vi "SiRealCenterFinder2Circles.vi"() -> ()   [LabVIEW 2019]
uses:
  <vilib>/userDefined/High Color/IMAQdx.ctl
  Other Models/2010/Motion/AbortSingle.vi
  <vilib>/vision/NI_Vision_Development_Module.lvlib
panel:
  in  "AutoFocus":bool
  in  "InitialStepSize":dbl=0.1 format="%#_13g"
  in  "AbortAutoFocus":bool
  in  "VisibilityInCamera":enum16{"JoyStick", "ClickToMove", "AllVisible"}(ring)
  out "UsedCoordinates":string
  in  "AdjustCamera":T1={"+Y"=FALSE, "-Z"=FALSE, "Done"=FALSE, "+Z"=FALSE, "-Y"=FALSE, "-X"=FALSE, "+X"=FALSE, "MoveXYBy(mm)"=0.25, "MoveZBy(mm)"=0.1} {"MoveZBy(mm)" format="%#_13g"}
  in  "StopJoyStick":bool
  out "CameraGcode":string
  in  "SiOnBPFiducials":path=path "C:/Users/TTUHEP/Documents/LabVIEW/GantryPrograms/Configs/SiOnBPFiducialsA1.txt"
  out "Dev":dbl
  out "ImageCurrent":T2(plugin-control)
  out "Image2":T2(plugin-control)
  out "Image1":T2(plugin-control)
  out "Output XYZU":string
  in  "HexaboardEdges":path=path "C:/Users/TTUHEP/Documents/LabVIEW/GantryPrograms/Configs/PCB1_4Points.txt"
  in  "SiFiducials":path=path "C:/Users/TTUHEP/Documents/LabVIEW/GantryPrograms/Utilities/WorkInProgress/SensorFids4At30deg.txt"
  in  "Component":enum16{"Baseplate", "Si", "SiOnBP", "PCB"}(ring)=enum."Si"
  in  "BasePlateEdges":path=path "C:/Users/TTUHEP/Documents/LabVIEW/GantryPrograms/Configs/Baseplate1CuPoints.txt"
  # "Use \"Si\" or \"SiOnBP\".\nNot supported: \"Baseplate\", \"PCB\""
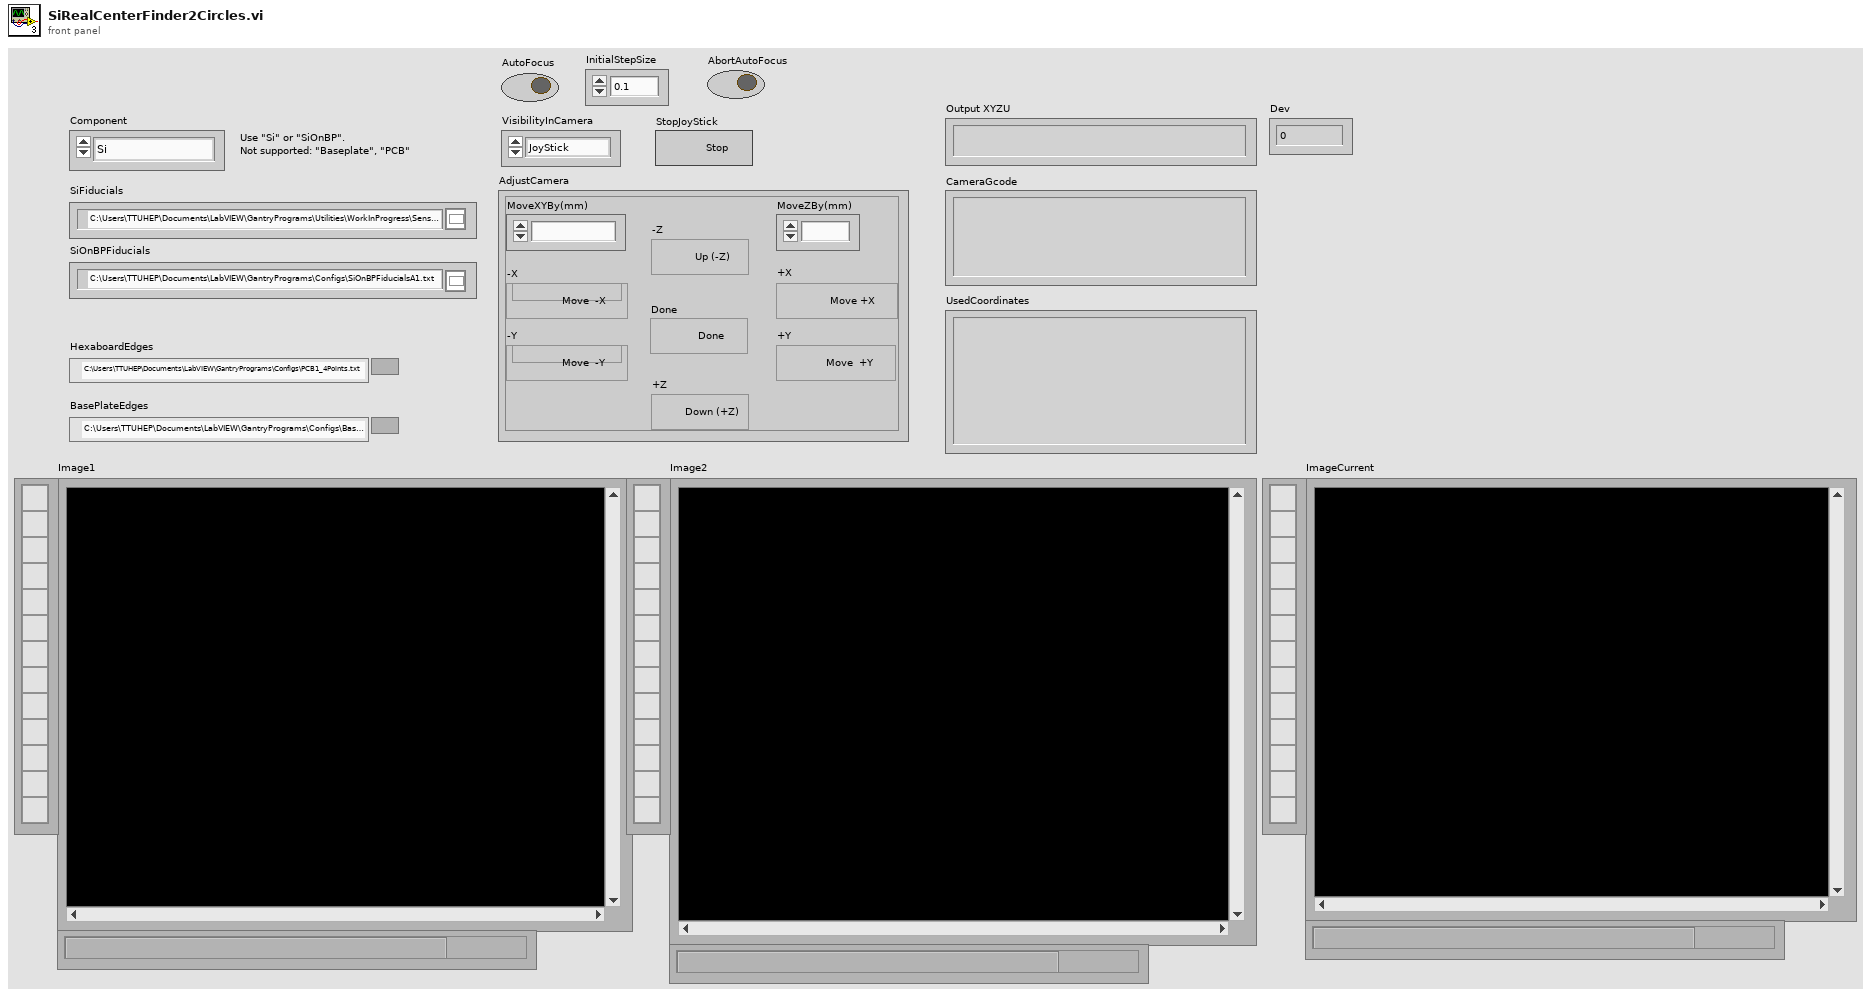
[diagram p1: front panel]
types:
  T1 = cluster{"+Y":bool, "-Z":bool, "Done":bool, "+Z":bool, "-Y":bool, "-X":bool, "+X":bool, "MoveXYBy(mm)":dbl, "MoveZBy(mm)":dbl}
  T2 = typedef "IMAQ Image.ctl" = refnum<image>
  T3 = typedef "IMAQdx.ctl" = refnum<k21>
  T4 = enum16{"Convolution", "Differentiation", "Gradient", "Prewitt", "Roberts", "Sigma", "Sobel"}
  T5 = typedef "Image Type" = u32
  T6 = cluster{"Position":cluster{"X":sgl, "Y":sgl}, "Radius":dbl, "Score":dbl}
  T7 = enum16{"Left Button", "Center Button", "Right Button", "Window Close"}
  T8 = enum16{"open", "replace", "create", "open or create", "replace or create", "replace or create with confirmation"}
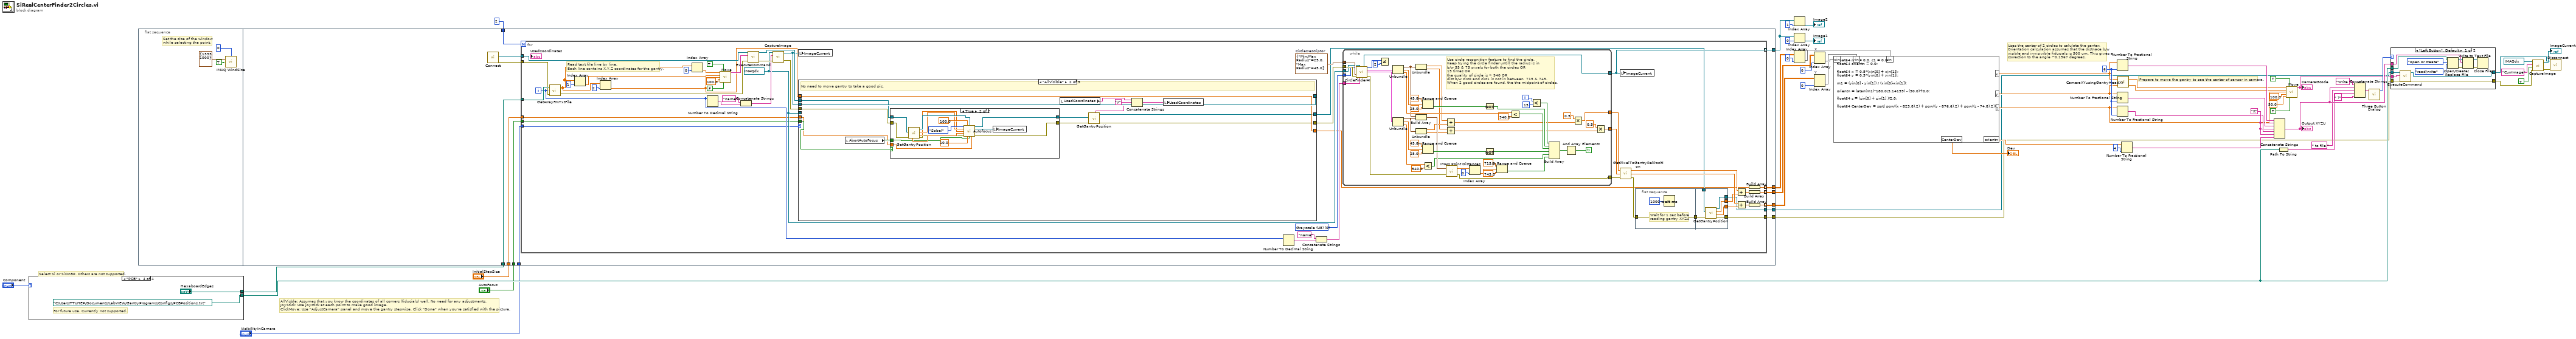
[diagram p0: block diagram]
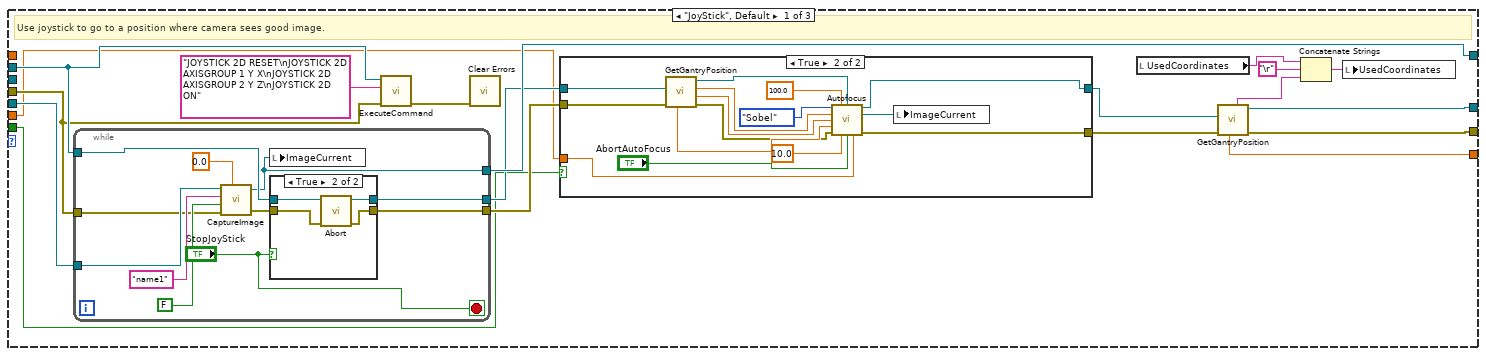
[diagram p3: hidden frame]
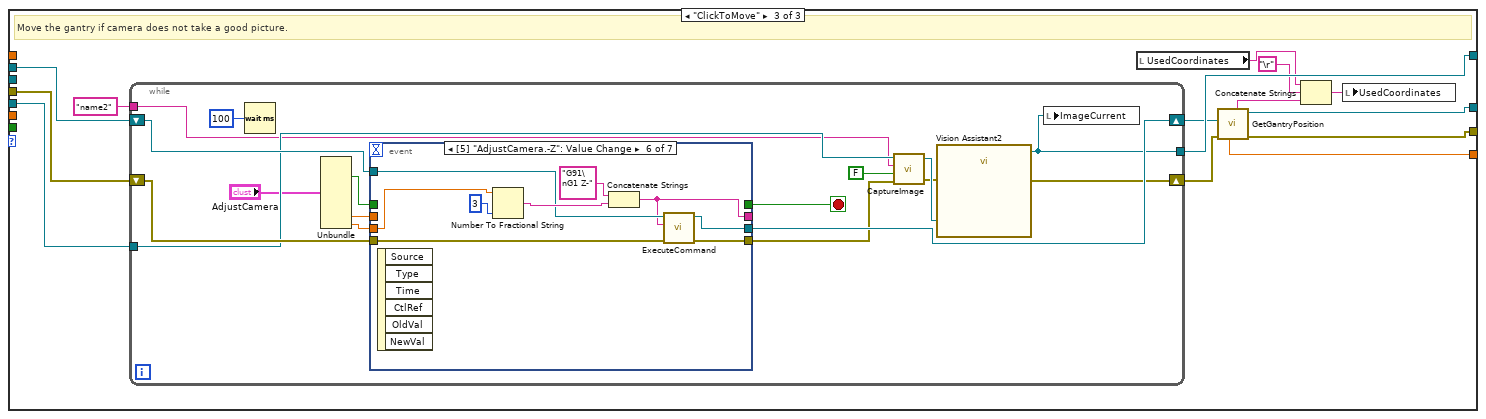
[diagram p7: hidden frame]
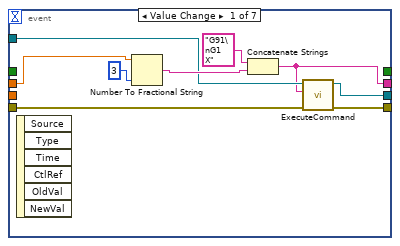
[diagram p8: hidden frame]
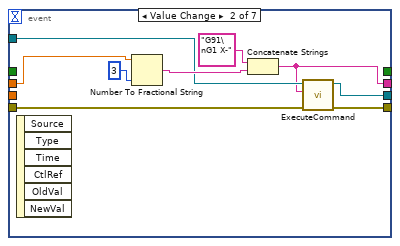
[diagram p9: hidden frame]
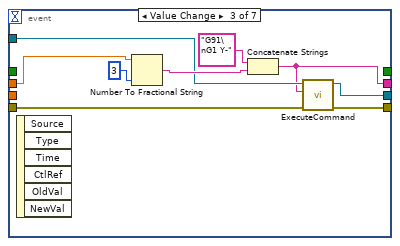
[diagram p10: hidden frame]
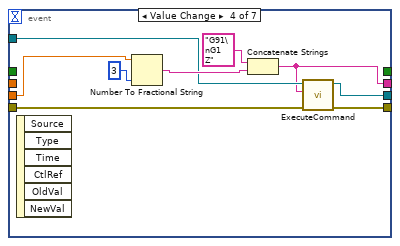
[diagram p11: hidden frame]
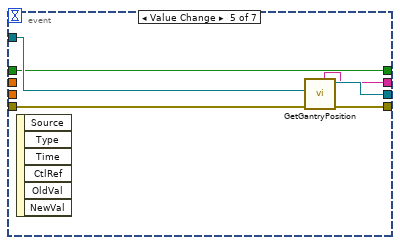
[diagram p12: hidden frame]
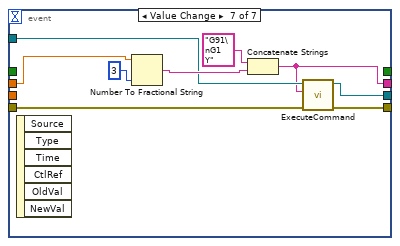
[diagram p13: hidden frame]
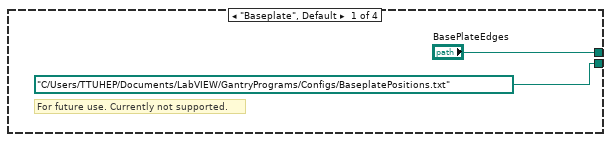
[diagram p14: hidden frame]
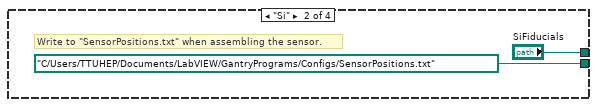
[diagram p15: hidden frame]
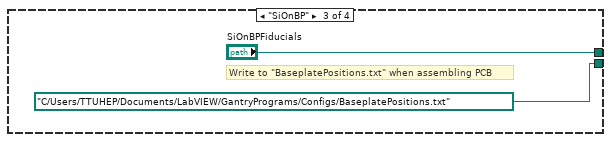
[diagram p16: hidden frame]
diagram:
  w52 = "\t"
  w49 = i16 6 ("width (-)")
  # "AllVisble: Assumes that you know the coordinates of all corners (fiducials) well. No need for any adjustments.\nJoyStick: Use joystick at each point to make good image.\nClickMove: Use \"AdjustCamera\" panel and move the gantry stepwise. Click \"Done\" when you're satisfied with the picture."
  # "Select Si or SiOnBP. Others are not supported."
  # "Prepare to move the gantry to see the center of sensor in camera."
  # "Uses the center of 2 circles to calulate the center.\nOrientation calculation assumes that the distnace b/w\nvisible and invisivible fiducials is 500 um. This gives a \ncorrection to the angle ~0.1567 degrees."
  n1 = case shown="\"PCB\"" "Component" {
    tunnel: ["BasePlateEdges" "SiFiducials" "SiOnBPFiducials" "HexaboardEdges"] -> w55
    tunnel: [path "C:/Users/TTUHEP/Documents/LabVIEW/GantryPrograms/Configs/BaseplatePositions.txt" ("OutFile") path "C:/Users/TTUHEP/Documents/LabVIEW/GantryPrograms/Configs/SensorPositions.txt" ("OutFile") path "C:/Users/TTUHEP/Documents/LabVIEW/GantryPrograms/Configs/BaseplatePositions.txt" ("OutFile") path "C:/Users/TTUHEP/Documents/LabVIEW/GantryPrograms/Configs/PCBPositions.txt" ("OutFile")] -> w40
    frame "Baseplate", Default {
      # "For future use. Currently not supported."
    }
    frame "Si" {
      # "Write to \"SensorPositions.txt\" when assembling the sensor."
    }
    frame "SiOnBP" {
      # "Write to \"BaseplatePositions.txt\" when assembling PCB"
    }
    frame "PCB" {
      # "For future use. Currently not supported."
    }
  }
  n2 = flat-sequence {
    tunnel: 2 -> [w80]
    tunnel: w55 -> [w79]
    tunnel: [w78] -> w11
    tunnel: [w77] -> w10
    tunnel: [w74] -> w22
    tunnel: [w73] -> w38
    tunnel: [w72] -> w1
    tunnel: [w71] -> w2
    tunnel: "VisibilityInCamera" -> [w70]
    tunnel: "AutoFocus" -> [w69]
    tunnel: "InitialStepSize" -> [w68]
    frame #0 {
      # "Set the size of the window\nwhile selecting the point."
      n3 = call "IMAQ WindSize"("Scrollbars? (N)"=TRUE, "Width & Height"=cluster{"Width":i32, "Height":i32} {"Width"=1333, "Height"=1000}, "Window Number"=0) -> ()  [unwired: 3 in, 3 out]
    }
    frame #1 {
      n4 = call "Connect.vi"() -> ("error out"=w76:errorcluster, "controller"=w75:refnum<k24>)  [unwired: 10 in]
      n5 = for {
        N: w80 -> [_]
        tunnel: w79 -> [w128]
        tunnel: w75 -> [w123]
        tunnel: w76 -> [w122]
        tunnel: [w102] -> w78
        tunnel: [w99] -> w77
        tunnel: [w103] -> w74 mode=indexing
        tunnel: [w118] -> w73 mode=indexing
        tunnel: [w117] -> w72 mode=indexing
        tunnel: [w116] -> w71 mode=indexing
        tunnel: w70 -> [w89]
        tunnel: w69 -> [w82]
        tunnel: w68 -> [w81]
        i -> [w93]
        w108 = cluster{"Min/Max Radius":dbl, "Max Radius":dbl} {"Min/Max Radius"=25.0, "Max Radius"=45.0}  # CircleDescriptor
        w91 = T3 "cam1" ("Session In")
        w107 = T5 0 items=["Grayscale (U8)", "Grayscale (I16)", "Grayscale (SGL)", "Complex (CSG)", "RGB (U32)", "HSL (U32)", "RGB (U64)", "Grayscale (U16)"] ("Image Type")
        # "Read text file line by line.\nEach line contains X,Y,Z coordinates for the gantry."
        n6 = call "GetArrayFmTxtFile.vi"("error in"=w122, "LineNo."=w93, "TextFile"=w128) -> ("error out"=w121:errorcluster, "Array"=w129:dbl[])
        n7 = Index Array(array=w129, index=1) -> (element=w112:dbl)
        n8 = Index Array(array=w129, index=2) -> (element=w83:dbl)
        n9 = Index Array(array=w129, index=0) -> (element=w114:dbl)
        n10 = Number To Decimal String(number=w93) -> (decimal integer string=w95:string)  [unwired: 1 in]
        n11 = call "Move.vi"("X"=w114, "Absolute"=TRUE, "Y"=w112, "Z"=w83, "SpeedXY (mm/s)"=100.0, "Move Z first"=FALSE) -> ("Position Gcode"=w124:string)  [unwired: 9 in]
        n12 = Concatenate Strings("name" ("string"), w95) -> (w92:string)
        n13 = call "ExecuteCommand.vi"("error in (no error)"=w121, "Command Code"=w124, "controller in"=w123) -> ("error out"=w96:errorcluster, "controller out"=w90:refnum<k24>)  [unwired: 6 in, 1 out]
        n14 = call "CaptureImage.vi"("Camera"=w91, "ImageName"=w92, "error in (no error)"=w96) -> ("Image"=w85:T2, "error out"=w86:errorcluster)  [unwired: 4 in]
        n15 = local write "ImageCurrent"(w85) -> ()
        n16 = case shown="\"AllVisible\"" w89 {
          tunnel: w91 -> [w150 _ w230]
          tunnel: w90 -> [w148 w197 w229]
          tunnel: w86 -> [w146 w195 w228]
          tunnel: [w149 w200 w227] -> _
          tunnel: [w145 w194 w219] -> w88
          tunnel: [w144 w191 w221] -> w87
          tunnel: w85 -> [_ w200 _]
          tunnel: [w139 w199 w218] -> w84
          tunnel: w83 -> [_ w199 _]
          tunnel: w82 -> [w134 w196 _]
          tunnel: w81 -> [w133 w186 _]
          frame "JoyStick", Default {
            # "Use joystick to go to a position where camera sees good image."
            n17 = while {
              tunnel: w150 -> [w178]
              tunnel: [w169] -> w149
              tunnel: w148 -> [w175]
              tunnel: [w172] -> w137
              tunnel: [w171] -> w138
              tunnel: w146 -> [w170]
              stop <- "StopJoyStick" stop-if-true
              n18 = call "CaptureImage.vi"("Camera"=w178, "Rotate (degrees)"=sgl 0.0, "ImageName"="name1", "Draw50MicroCircleAtCenter"=FALSE, "error in (no error)"=w170) -> ("Image"=w169:T2, "error out"=w173:errorcluster)  [unwired: 2 in]
              n19 = local write "ImageCurrent"(w169) -> ()
              n20 = case shown="True" "StopJoyStick" {
                tunnel: w175 -> [w181 w185]
                tunnel: w173 -> [w180 w184]
                tunnel: [w180 w183] -> w172
                tunnel: [w181 w182] -> w171
                frame False {
                }
                frame True {
                  n21 = call-poly "Abort.vi"("error in (no error)"=w184, "controller in"=w185) -> ("error out"=w183:errorcluster, "controller out"=w182:refnum<k24>)  [unwired: 8 in]
                }
              }
            }
            n22 = call "ExecuteCommand.vi"("error in (no error)"=w146, "Command Code"="JOYSTICK 2D RESET\nJOYSTICK 2D AXISGROUP 1 Y X\nJOYSTICK 2D AXISGROUP 2 Y Z\nJOYSTICK 2D ON", "controller in"=w148) -> ("error out"=w147:errorcluster)  [unwired: 6 in, 2 out]
            n23 = call <vilib>:"Clear Errors.vi"("error in (no error)"=w147) -> ()  [unwired: 5 in, 2 out]
            n24 = case shown="True" w134 {
              tunnel: w138 -> [w153 w168]
              tunnel: w137 -> [w152 w167]
              tunnel: [w153 w157] -> w136
              tunnel: [w152 w156] -> w135
              tunnel: w133 -> [_ w154]
              frame False {
              }
              frame True {
                n25 = call "GetGantryPosition.vi"("error in (no error)"=w167, "Controller In"=w168) -> ("error out"=w160:errorcluster, "Position Y"=w162:dbl, "Position X"=w163:dbl, "controller out"=w166:refnum<k24>, "Position Z"=w161:dbl)  [unwired: 3 in, 2 out]
                n26 = call "Autofocus.vi"("SafeMaxZ"=T4."Sobel" ("Filter Type"), "SpeedXY (mm/s)"=100.0, "controller in"=w166, "X"=w163, "Y"=w162, "Z"=w161, "error in (no error)"=w160, "SpeedZ (mm/s)"=10.0, "AbortAutoFocus"="AbortAutoFocus", "InitialStepSize"=w154) -> ("controller out"=w157:refnum<k24>, "Image"=w155:T2, "error out"=w156:errorcluster)  [unwired: 1 in, 2 out]
                n27 = local write "ImageCurrent"(w155) -> ()
              }
            }
            n28 = local read "UsedCoordinates"() -> (w142:string)
            n29 = call "GetGantryPosition.vi"("error in (no error)"=w135, "Controller In"=w136) -> ("error out"=w144:errorcluster, "controller out"=w145:refnum<k24>, "Position_XYZ"=w140:string, "Position Z"=w139:dbl)  [unwired: 3 in, 3 out]
            n30 = Concatenate Strings(w142, "\r", w140) -> (w143:string)
            n31 = local write "UsedCoordinates"(w143) -> ()
          }
          frame "AllVisible" {
            # "No need to move gantry to take a good pic."
            n32 = local read "AbortAutoFocus"() -> (w187:bool)
            n33 = case shown="True" w196 {
              tunnel: w197 -> [w202 w210]
              tunnel: w195 -> [w201 w209]
              tunnel: [w201 w205] -> w192
              tunnel: [w202 w208] -> w193
              tunnel: w187 -> [_ w204]
              tunnel: w186 -> [_ w203]
              frame False {
              }
              frame True {
                n34 = call "GetGantryPosition.vi"("error in (no error)"=w209, "Controller In"=w210) -> ("error out"=w206:errorcluster, "Position Y"=w213:dbl, "Position X"=w214:dbl, "controller out"=w217:refnum<k24>, "Position Z"=w212:dbl)  [unwired: 3 in, 2 out]
                n35 = call "Autofocus.vi"("SafeMaxZ"=T4."Sobel" ("Filter Type"), "SpeedXY (mm/s)"=100.0, "controller in"=w217, "X"=w214, "Y"=w213, "Z"=w212, "error in (no error)"=w206, "SpeedZ (mm/s)"=10.0, "AbortAutoFocus"=w204, "InitialStepSize"=w203) -> ("controller out"=w208:refnum<k24>, "Image"=w207:T2, "error out"=w205:errorcluster)  [unwired: 1 in, 2 out]
                n36 = local write "ImageCurrent"(w207) -> ()
              }
            }
            n37 = local read "UsedCoordinates"() -> (w189:string)
            n38 = call "GetGantryPosition.vi"("error in (no error)"=w192, "Controller In"=w193) -> ("error out"=w191:errorcluster, "controller out"=w194:refnum<k24>, "Position_XYZ"=w188:string)  [unwired: 3 in, 4 out]
            n39 = Concatenate Strings(w189, "\r", w188) -> (w190:string)
            n40 = local write "UsedCoordinates"(w190) -> ()
          }
          frame "ClickToMove" {
            # "Move the gantry if camera does not take a good picture."
            n41 = while {
              shift-right: [w240] -> w222
              shift-left: w228 -> [w248]
              shift-right: [w246] -> w220
              shift-left: w229 -> [w247]
              tunnel: "name2" ("ImageName") -> [w242]
              tunnel: w230 -> [w243]
              tunnel: [w232] -> w227
              stop <- w245 stop-if-true
              n42 = Wait (ms)(milliseconds to wait=u32 100) -> ()  [unwired: 1 out]
              n43 = Unbundle("AdjustCamera") -> ("Done"=w236:bool, "MoveXYBy(mm)"=w234:dbl, "MoveZBy(mm)"=w235:dbl)  [unwired: 6 out]
              n44 = event shown="[5] \"AdjustCamera.-Z\": Value Change" {
                selector: _ -> [_ _ _ _ _ _ _]
                dyn-events: _ -> [_ _ _ _ _ _ _]
                timeout: _ -> [_ _ _ _ _ _ _]
                tunnel: w234 -> [w254 w258 w267 _ _ _ w300]
                tunnel: w248 -> [w253 w262 w271 w280 w289 w295 w304]
                tunnel: [w252 w261 w270 w277 w286 w294 w303] -> w241
                tunnel: w247 -> [w251 w263 w272 w281 w290 w296 w305]
                tunnel: [w250 w260 w269 w278 w288 w293 w302] -> w246
                tunnel: [w249 w259 w268 w279 w287 w292 w301] -> _
                tunnel: [_ _ _ _ w285 _ _] -> w245
                tunnel: w235 -> [_ _ _ w276 _ w291 _]
                tunnel: w236 -> [_ _ _ _ w285 _ _]
                event "AdjustCamera.+X": Value Change {
                  n45 = event-data() -> ()  [unwired: 1 in, 6 out]
                  n46 = Number To Fractional String(number=w254, precision (6)=3) -> (F-format string=w257:string)  [unwired: 2 in]
                  n47 = Concatenate Strings("G91\nG1 X", w257) -> (w249:string)
                  n48 = call "ExecuteCommand.vi"("error in (no error)"=w253, "Command Code"=w249, "controller in"=w251) -> ("error out"=w252:errorcluster, "controller out"=w250:refnum<k24>)  [unwired: 6 in, 1 out]
                }
                event "AdjustCamera.-X": Value Change {
                  n49 = event-data() -> ()  [unwired: 1 in, 6 out]
                  n50 = Number To Fractional String(number=w258, precision (6)=3) -> (F-format string=w266:string)  [unwired: 2 in]
                  n51 = Concatenate Strings("G91\nG1 X-", w266) -> (w259:string)
                  n52 = call "ExecuteCommand.vi"("error in (no error)"=w262, "Command Code"=w259, "controller in"=w263) -> ("error out"=w261:errorcluster, "controller out"=w260:refnum<k24>)  [unwired: 6 in, 1 out]
                }
                event "AdjustCamera.-Y": Value Change {
                  n53 = event-data() -> ()  [unwired: 1 in, 6 out]
                  n54 = Number To Fractional String(number=w267, precision (6)=3) -> (F-format string=w275:string)  [unwired: 2 in]
                  n55 = Concatenate Strings("G91\nG1 Y-", w275) -> (w268:string)
                  n56 = call "ExecuteCommand.vi"("error in (no error)"=w271, "Command Code"=w268, "controller in"=w272) -> ("error out"=w270:errorcluster, "controller out"=w269:refnum<k24>)  [unwired: 6 in, 1 out]
                }
                event "AdjustCamera.+Z": Value Change {
                  n57 = event-data() -> ()  [unwired: 1 in, 6 out]
                  n58 = Number To Fractional String(number=w276, precision (6)=3) -> (F-format string=w284:string)  [unwired: 2 in]
                  n59 = Concatenate Strings("G91\nG1 Z", w284) -> (w279:string)
                  n60 = call "ExecuteCommand.vi"("error in (no error)"=w280, "Command Code"=w279, "controller in"=w281) -> ("error out"=w277:errorcluster, "controller out"=w278:refnum<k24>)  [unwired: 6 in, 1 out]
                }
                event "AdjustCamera.Done": Value Change {
                  n61 = event-data() -> ()  [unwired: 1 in, 6 out]
                  n62 = call "GetGantryPosition.vi"("error in (no error)"=w289, "Controller In"=w290) -> ("error out"=w286:errorcluster, "controller out"=w288:refnum<k24>, "Position_XYZ"=w287:string)  [unwired: 3 in, 4 out]
                }
                event "AdjustCamera.-Z": Value Change {
                  n63 = event-data() -> ()  [unwired: 1 in, 6 out]
                  n64 = Number To Fractional String(number=w291, precision (6)=3) -> (F-format string=w299:string)  [unwired: 2 in]
                  n65 = Concatenate Strings("G91\nG1 Z-", w299) -> (w292:string)
                  n66 = call "ExecuteCommand.vi"("error in (no error)"=w295, "Command Code"=w292, "controller in"=w296) -> ("error out"=w294:errorcluster, "controller out"=w293:refnum<k24>)  [unwired: 6 in, 1 out]
                }
                event "AdjustCamera.+Y": Value Change {
                  n67 = event-data() -> ()  [unwired: 1 in, 6 out]
                  n68 = Number To Fractional String(number=w300, precision (6)=3) -> (F-format string=w308:string)  [unwired: 2 in]
                  n69 = Concatenate Strings("G91\nG1 Y", w308) -> (w301:string)
                  n70 = call "ExecuteCommand.vi"("error in (no error)"=w304, "Command Code"=w301, "controller in"=w305) -> ("error out"=w303:errorcluster, "controller out"=w302:refnum<k24>)  [unwired: 6 in, 1 out]
                }
              }
              n71 = call "CaptureImage.vi"("Camera"=w243, "ImageName"=w242, "Draw50MicroCircleAtCenter"=FALSE, "error in (no error)"=w241) -> ("Image"=w239:T2, "error out"=w238:errorcluster)  [unwired: 3 in]
              n72 = call "Vision Assistant2"("Image In"=w239, "error in"=w238) -> ("Image Out"=w232:T2, "error out"=w240:errorcluster)  [unwired: 24 in]
              n73 = local write "ImageCurrent"(w232) -> ()
            }
            n74 = local read "UsedCoordinates"() -> (w225:string)
            n75 = call "GetGantryPosition.vi"("error in (no error)"=w222, "Controller In"=w220) -> ("error out"=w221:errorcluster, "controller out"=w219:refnum<k24>, "Position_XYZ"=w223:string, "Position Z"=w218:dbl)  [unwired: 3 in, 3 out]
            n76 = Concatenate Strings(w225, "\r", w223) -> (w226:string)
            n77 = local write "UsedCoordinates"(w226) -> ()
          }
        }
        n78 = Number To Decimal String(number=w93) -> (decimal integer string=w120:string)  [unwired: 1 in]
        n79 = Concatenate Strings("name" ("string"), w120) -> (w109:string)
        n80 = while {
          tunnel: w109 -> [w349]
          tunnel: w91 -> [w353]
          tunnel: w108 -> [w354]
          tunnel: w107 -> [w350]
          tunnel: [w336] -> w106
          tunnel: [w352] -> w103
          tunnel: [w318] -> w105
          tunnel: [w317] -> w104
          tunnel: w87 -> [w355]
          i -> [w368]
          stop <- w356 continue-if-true
          # "Use circle recognition feature to find the circle.\nKeep trying the circle finder untill the radius is in \nb/w 55 & 75 pixels for both the circles OR\n15 times OR\nthe quality of circle is > 940 OR\ndist b/w circ0 and circ1 is not in between  715 & 745.\nWhen 2 good circles are found, the the midpoint of circles."
          n81 = call "CircleFinderAI.vi"("Image Type"=w350, "Session In"=w353, "Circle Descriptor"=w354, "error in (no error)"=w355, "Image Name"=w349) -> ("Image"=w352:T2, "NumCirclesFound"=w348:i32, "Circle0"=w351:T6, "Circle1"=w346:T6, "error out"=w337:errorcluster)  [unwired: 5 in, 1 out]
          n82 = Not Equal?(x=w348, y=2) -> ()  [unwired: 1 out]
          n83 = Unbundle(w351) -> ("Position"=w339:cluster{"X":sgl, "Y":sgl}, "Radius"=w362:dbl, "Score"=w366:dbl)
          n84 = Unbundle(w346) -> ("Position"=w326:cluster{"X":sgl, "Y":sgl}, "Radius"=w341:dbl, "Score"=w340:dbl)
          n85 = Unbundle(w339) -> ("X"=w327:sgl, "Y"=w320:sgl)
          n86 = Build Array(w339, w326) -> (w338:cluster{"X":sgl, "Y":sgl}[])
          n87 = Unbundle(w326) -> ("X"=w325:sgl, "Y"=w319:sgl)
          n88 = In Range and Coerce(upper limit=45.0, x=w362, lower limit=25.0) -> (In Range?=w361:bool)  [unwired: 1 out]
          n89 = In Range and Coerce(upper limit=45.0, x=w341, lower limit=25.0) -> (In Range?=w342:bool)  [unwired: 1 out]
          n90 = Less?(x=w340, y=940.0) -> (x < y?=w332:bool)
          n91 = Add(x=w327, y=w325) -> (x+y=w323:sgl)
          n92 = Add(x=w320, y=w319) -> (x+y=w321:sgl)
          n93 = call "IMAQ Point Distances"("Points"=w338, "error in (no error)"=w337) -> ("Distances"=w335:sgl[], "error out"=w336:errorcluster)  [unwired: 3 in]
          n94 = Index Array(array=w335, index=0) -> (element=w331:sgl)
          n95 = Not(x=w361) -> (.not. x?=w359:bool)
          n96 = Not(x=w342) -> (.not. x?=w333:bool)
          n97 = In Range and Coerce(upper limit=sgl 715.0, x=w331, lower limit=sgl 745.0) -> (In Range?=w328:bool)  [unwired: 1 out]
          n98 = Less?(x=w366, y=940.0) -> (x < y?=w358:bool)
          n99 = Less?(x=w368, y=15) -> (x < y?=w360:bool)
          n100 = Build Array(w360, w359, w358, w333, w332, w328) -> (w357:bool[])
          n101 = And Array Elements(Boolean array=w357) -> (logical AND=w356:bool)
          n102 = Multiply(x=0.5, y=w323) -> (x*y=w318:dbl)
          n103 = Multiply(x=0.5, y=w321) -> (x*y=w317:dbl)
        }
        n104 = local write "ImageCurrent"(w103) -> ()
        n105 = call "GetPixelToGantryRelPosition.vi"("error in (no error)"=w106, "PixelY"=w104, "PixelX"=w105) -> ("error out"=w97:errorcluster, "YmmRelGH"=w111:dbl, "XmmRelGH"=w115:dbl)
        n106 = flat-sequence {
          tunnel: [w309] -> w98
          tunnel: w97 -> [w309]
          tunnel: w88 -> [w316]
          tunnel: [w315] -> w102
          tunnel: [w314] -> w101
          tunnel: [w313] -> w100
          tunnel: [w312] -> w99
          tunnel: w98 -> [w311]
          frame #0 {
            # "Wait for 1 sec before\nreading gantry XYZU"
            n107 = Wait (ms)(milliseconds to wait=u32 1000) -> ()  [unwired: 1 out]
          }
          frame #1 {
            n108 = call "GetGantryPosition.vi"("error in (no error)"=w311, "Controller In"=w316) -> ("error out"=w315:errorcluster, "Position Y"=w314:dbl, "Position X"=w313:dbl, "controller out"=w312:refnum<k24>)  [unwired: 3 in, 3 out]
          }
        }
        n109 = Add(x=w115, y=w100) -> (x+y=w113:dbl)
        n110 = Add(x=w111, y=w101) -> (x+y=w110:dbl)
        n111 = Build Array(w84) -> (w118:dbl[])
        n112 = Build Array(w113) -> (w116:dbl[])
        n113 = Build Array(w110) -> (w117:dbl[])
      }
    }
  }
  n114 = Index Array(array=w22, index=1 ("length")) -> (element=→"Image2":T2)
  n115 = Index Array(array=w22, index=0 ("length")) -> (element=→"Image1":T2)
  n116 = Index Array(array=w38, index (col)=0 ("disabled index (col)")) -> (element=w28:dbl[])  [unwired: 1 in]
  n117 = Index Array "X"(array=w2, index (col)=0 ("disabled index (col)")) -> (element=w30:dbl[])  [unwired: 1 in]
  n118 = Index Array "Y"(array=w1, index (col)=0 ("disabled index (col)")) -> (element=w29:dbl[])  [unwired: 1 in]
  n119 = formula code="float64 m1 = 0.0, c1 = 0.0;\nfloat64 orientn = 0.0;\n\nfloat64 x = 0.5*(xin[0] + xin[1]); \nfloat64 y = 0.5*(yin[0] + yin[1]);\n\nm1 = (yin[0] - yin[1]) / (xin[0]-xin[1]);\n\norientn = (atan(m1)*180.0/3.14159) - (30.0)+0.0;\n\nfloat64 z = (zin[0] + zin[1] )/2.0;\n\nfloat64 CenterDev = sqrt( pow((x - 823.8),2) + pow((y - 876.6),2) + pow((z - 74.8),2));"("xin"=w30, "yin"=w29, "zin"=w28) -> ("orientn"=w27:dbl, "x"=w16:dbl, "y"=w13:dbl, "z"=w12:dbl, "CenterDev"=→"Dev":dbl)
  n120 = Number To Fractional String(number=w16, precision (6)=w49) -> (F-format string=w54:string)  [unwired: 2 in]
  n121 = Number To Fractional String(number=w13, precision (6)=w49) -> (F-format string=w53:string)  [unwired: 2 in]
  n122 = Number To Fractional String(number=w12, precision (6)=w49) -> (F-format string=w48:string)  [unwired: 2 in]
  n123 = call "CameraXYusingGantryHeadXY.vi"("GantryY"=w13, "GantryX"=w16) -> ("CamY"=w14:dbl, "CamX"=w15:dbl)
  n124 = Number To Fractional String(number=w27, precision (6)=i16 4 ("width (-)")) -> (F-format string=w50:string)  [unwired: 2 in]
  n125 = Concatenate Strings(w54, w52, w53, w52, w48, w52, w50) -> (w46:string)
  "Output XYZU" <- w46
  n126 = Path To String(path=w40) -> (string=w44:string)
  n127 = call "Move.vi"("X"=w15, "Absolute"=TRUE, "Y"=w14, "Z"=w12, "SpeedXY (mm/s)"=100.0, "SpeedZ (mm/s)"=50.0, "Move Z first"=TRUE) -> ("Position Gcode"=w7:string)  [unwired: 8 in]
  "CameraGcode" <- w7
  n128 = Concatenate Strings("Write ", w46, " to file ", w44, " ?" ("string")) -> (w42:string)
  n129 = call <vilib>:"Three Button Dialog.vi"("message"=w42) -> ("Which Button?"=w41:T7)  [unwired: 10 in]
  n130 = case shown="\"Left Button\", Default" w41 {
    tunnel: w46 -> [w375 _]
    tunnel: w40 -> [w374 _]
    tunnel: w11 -> [w373 w382]
    tunnel: w7 -> [w372 _]
    tunnel: w10 -> [w371 w383]
    tunnel: [w370 w382] -> w9
    tunnel: [w369 w383] -> w8
    frame "Left Button", Default {
      n131 = call "ExecuteCommand.vi"("error in (no error)"=w373, "Command Code"=w372, "controller in"=w371) -> ("error out"=w370:errorcluster, "controller out"=w369:refnum<k24>)  [unwired: 6 in, 1 out]
      n132 = Open/Create/Replace File(file path (use dialog)=w374, operation (0:open)=T8."open or create", access (0:read/write)=enum16{"read/write", "read-only", "write-only"}."read/write") -> (refnum out=w381:refnum<file>, error out=w378:errorcluster)  [unwired: 3 in, 1 out]
      n133 = Write to Text File(file (use dialog)=w381, text=w375, error in=w378) -> (refnum out=w376:refnum<file>, error out=w377:errorcluster)  [unwired: 1 in, 1 out]
      n134 = Close File(refnum=w376, error in=w377) -> ()  [unwired: 2 out]
    }
    frame "Center Button" {
    }
  }
  n135 = call "CaptureImage.vi"("Camera"=T3 "cam1", "ImageName"="CurrImage", "Draw50MicroCircleAtCenter"=TRUE, "error in (no error)"=w9) -> ("Image"=→"ImageCurrent":T2, "error out"=w21:errorcluster)  [unwired: 3 in]
  n136 = call "Disconnect.vi"("error in (no error)"=w21, "controller"=w8) -> ()  [unwired: 9 in, 1 out]
